vi "password validator.vi"(8 "error in":errorcluster, 10 "User Input":string, 11 "Users data":T2) -> (0 "error out":errorcluster, 1 "Full Name":string, 2 "Message out":T1, 3 "Users data out":T2)   [LabVIEW 2015]
uses:
  Controls/Users data.ctl
  Controls/user.ctl
  Controls/message.ctl
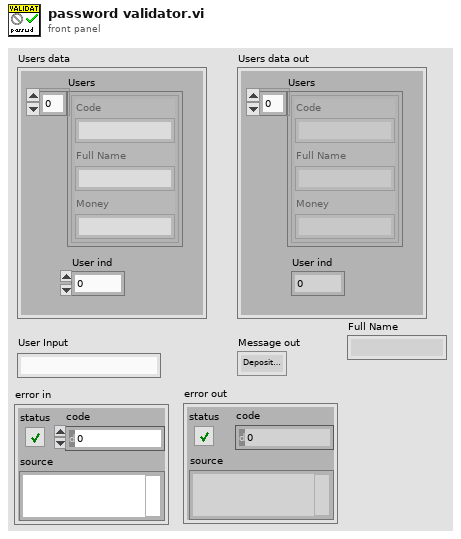
[diagram p1: front panel]
types:
  T1 = typedef "message.ctl" = enum16{"Deposit Complete", "Welcome", "Menu", "Verification Failed", "Session Terminate", "Deposit", "Withdrawal", "Withdrawal Complete", "Withdrawal Failed", "Balance Inq"}
  T2 = typedef "Users data.ctl" = cluster{"Users ":T3[], "User ind":i32}
  T3 = typedef "user.ctl" = cluster{"Full Name":string, "Code":string, "Money":string}
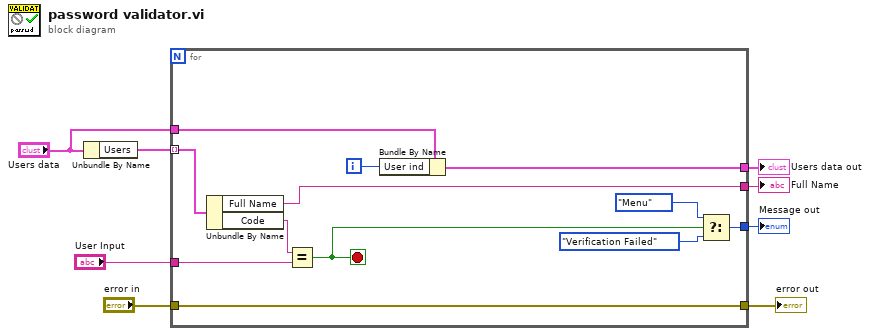
[diagram p0: block diagram]
diagram:
  n1 = Unbundle By Name("Users data") -> ("Users"=w4:T3[])
  n2 = for {
    tunnel: w4 -> [w10] mode=indexing
    tunnel: "User Input" -> [w19]
    tunnel: "Users data" -> [w18]
    tunnel: [w16] -> w7
    tunnel: [w12] -> w8
    tunnel: "error in" -> [w11]
    tunnel: [w11] -> w2
    tunnel: [w9] -> w1
    i -> [w17]
    stop <- w15 stop-if-true
    n3 = Unbundle By Name(w10) -> ("Full Name"=w9:string, "Code"=w20:string)
    n4 = Equal?(x=w20, y=w19) -> (x = y?=w15:bool)
    n5 = Bundle By Name(cluster=w18, "User ind"=w17) -> (w16:T2)
    n6 = Select(t=message."Menu" ("Message in"), s=w15, f=message."Verification Failed" ("Message in")) -> (s? t:f=w12:T1)
  }
  "Users data out" <- w7
  "Message out" <- w8
  "error out" <- w2
  "Full Name" <- w1
